vi "LM call model function gradient.vi"(5 "grad( f(x,a) )":T2, 7 "function data":T1, 8 "error in (no error)":errorcluster, 11 "a":dbl[](array[numeric])) -> (0 "error out":errorcluster, 3 "f(X)":dbl[][](array[numeric]))   [LabVIEW 2020, in "NI_Gmath.lvlib"]
uses:
  NI_Gmath.lvlib
  LM model function gradient reference.ctl
  objective function data.ctl
panel:
  in  "X":dbl[](array[numeric])
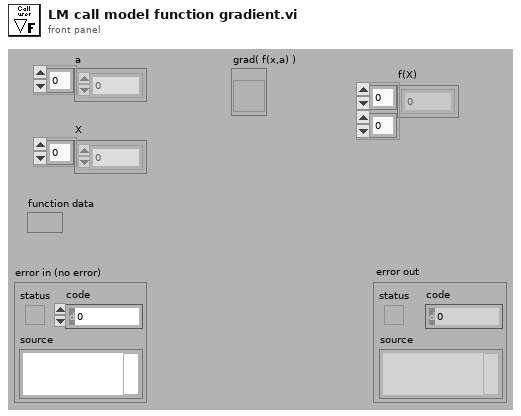
[diagram p1: front panel]
types:
  T1 = typedef "NI_Gmath.lvlib/objective function data.ctl" = variant
  T2 = typedef "NI_Gmath.lvlib/LM model function gradient reference.ctl" = refnum<vi>
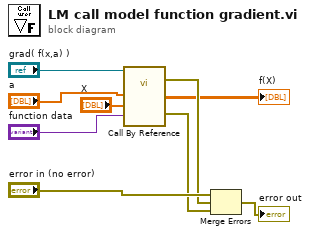
[diagram p0: block diagram]
diagram:
  n1 = call-by-ref "?"(reference="grad( f(x,a) )", "Variant"="function data", "Array 2"="X", "Array"="a") -> (error out=w6:errorcluster, 0:"error out"=w2:errorcluster, "Array 3"=→"f(X)":dbl[][])  [unwired: 1 in, 1 out]
  n2 = Merge Errors("error in (no error)", w6, w2) -> (→"error out":errorcluster)
